vi "PromptForProjNum.vi"(1 "project":string caption="ProjectNumber") -> (0 "ProjectNumber OUT":string caption="ProjectNumber")   [LabVIEW 2021]
doc: "Displays a standard dialog box that prompts users to enter information, such as a user name and password.\n--------------------\n\nThis Express VI is configured as follows:\n\nMessage to Display to the User:Project Number is required in order to file results correctly. Please enter the Project Number\nThe inputs are: \nText Entry Box: ProjectNumber"
uses:
  Globals/Constants_global.vi
panel:
  in  "existing":bool
  out "End":bool
  out "Startup":bool
  in  "OK":bool caption="OK1"
  # "Project Folder Name is required in order to file results correctly.\n\nPlease Accept , Update, or Browse for the Project Folder.  :"
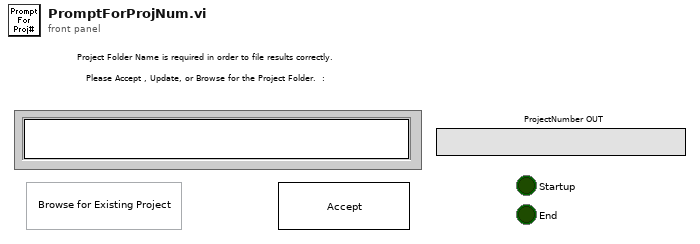
[diagram p1: front panel]
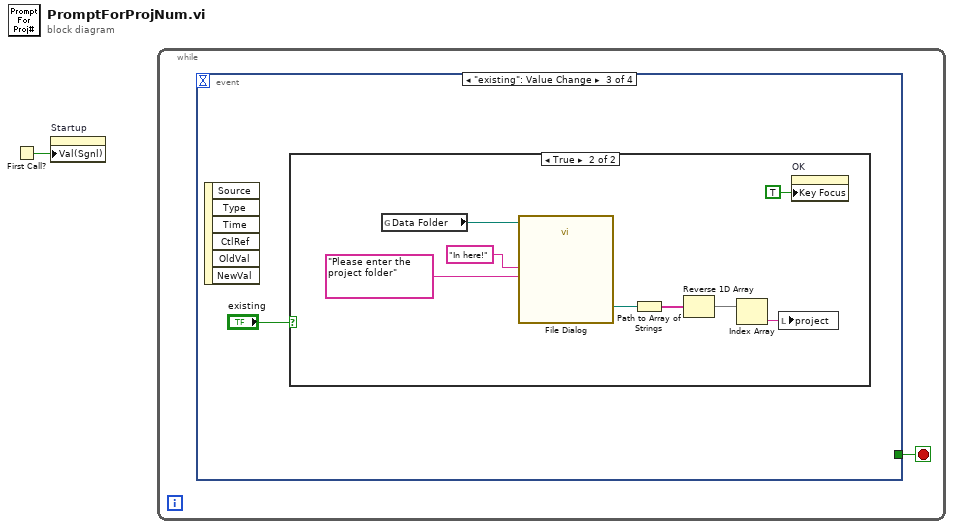
[diagram p0: block diagram]
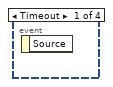
[diagram p2: hidden frame]
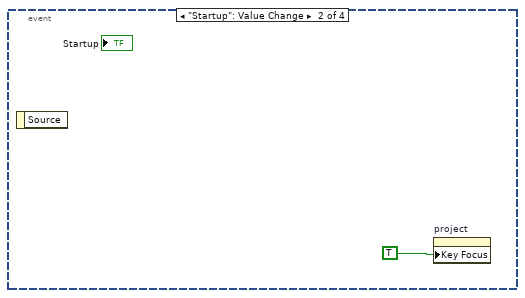
[diagram p3: hidden frame]
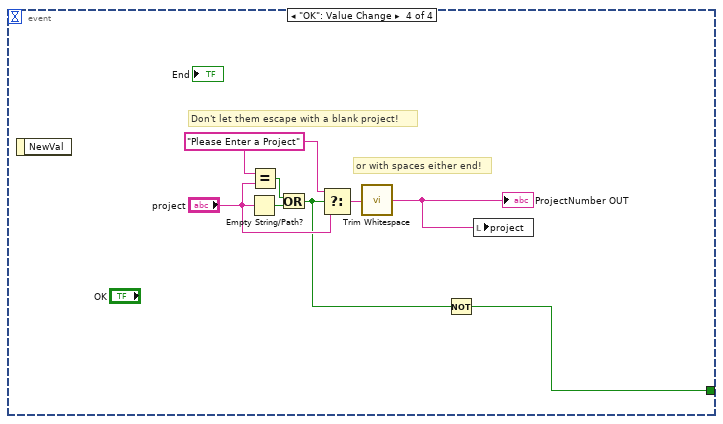
[diagram p5: hidden frame]
diagram:
  n1 = First Call?() -> (First Call?: T/F=w1:bool)
  n2 = property on="Startup" class="Bool (strict)"("Val(Sgnl)"=w1) -> ()  [unwired: 2 in, 2 out]
  n3 = while {
    stop <- w2 stop-if-true
    n4 = event shown="[2] \"existing\": Value Change" {
      selector: _ -> [_ _ _ _]
      dyn-events: _ -> [_ _ _ _]
      timeout: _ -> [_ _ _ _]
      tunnel: [_ _ _ w19] -> w2
      event Timeout {
        n5 = event-data() -> ()  [unwired: 1 in, 1 out]
      }
      event "Startup": Value Change {
        n6 = event-data() -> ()  [unwired: 1 in, 1 out]
        n7 = property on="project" class="Str"("Key Focus"=TRUE ("focus on")) -> ()  [unwired: 2 in, 2 out]
      }
      event "existing": Value Change {
        n8 = event-data() -> ()  [unwired: 1 in, 6 out]
        n9 = case shown="True" "existing" {
          frame False {
          }
          frame True {
            n10 = global read "Constants_global.vi" "Data Folder"() -> (w5:path)
            n11 = call "File Dialog"("start path"=w5, "prompt"="Please enter the project folder", "button label"="In here!") -> ("selected path"=w10:path)  [unwired: 9 in, 3 out]
            n12 = Path to Array of Strings(0:w10) -> (2:w9:string[])  [unwired: 1 out]
            n13 = Reverse 1D Array(array=w9) -> (reversed array=w6:string[])
            n14 = Index Array(array=w6) -> (element=w8:string)  [unwired: 1 in]
            n15 = local write "project"(w8) -> ()
            n16 = property on="OK" class="Bool"("Key Focus"=TRUE ("OK")) -> ()  [unwired: 2 in, 2 out]
          }
        }
      }
      event "OK": Value Change {
        w16 = "Please Enter a Project" ("t")
        # "or with spaces either end!"
        # "Don't let them escape with a blank project!"
        n17 = event-data() -> ()  [unwired: 1 in, 1 out]
        n18 = Empty String/Path?(string/path="project") -> (empty?=w20:bool)
        n19 = Equal?(x=w16, y="project") -> (x = y?=w14:bool)
        n20 = Or(x=w14, y=w20) -> (x .or. y?=w15:bool)
        n21 = Select(t=w16, s=w15, f="project") -> (s? t:f=w18:string)
        n22 = call <vilib>:"Trim Whitespace.vi"("string"=w18) -> ("trimmed string"=w13:string)  [unwired: 1 in]
        "ProjectNumber OUT" <- w13
        n23 = Not(x=w15) -> (.not. x?=w19:bool)
        n24 = local write "project"(w13) -> ()
      }
    }
  }
